vi "Drive Station HUD.vi"() -> ()   [LabVIEW 2018]
uses:
  <vilib>/vision/NI_Vision_Development_Module.lvlib
panel:
  out "Final Image":T1(plugin-control)
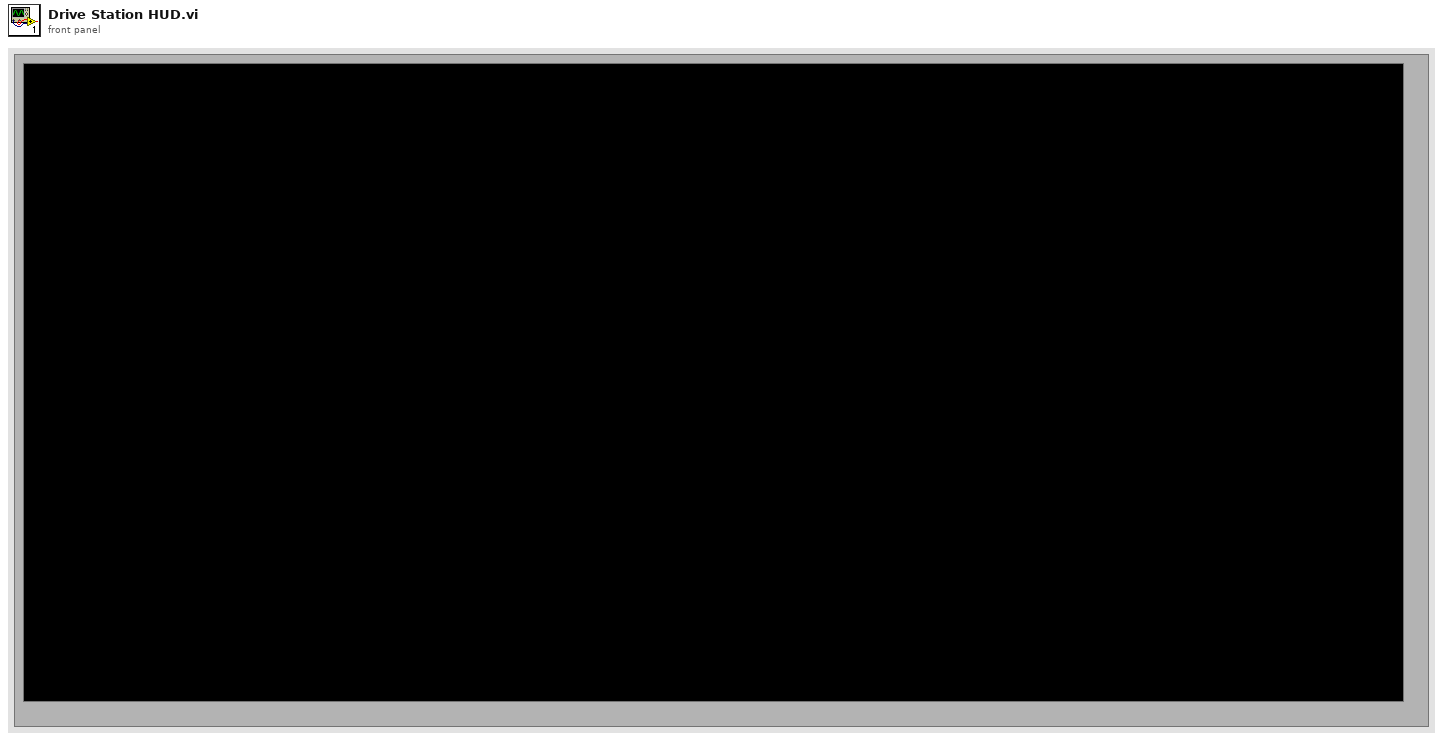
[diagram p1: front panel]
types:
  T1 = typedef "IMAQ Image.ctl" = refnum<image>
  T2 = typedef "Image Type" = u32
  T3 = typedef "LVAllMonitorsDisplayTypeDef.ctl" = cluster{"Bounds":cluster{"Left":i16, "Top":i16, "Right":i16, "Bottom":i16}, "Depth":i16}[]
  T4 = cluster{"Left":i16, "Top":i16, "Right":i16, "Bottom":i16}
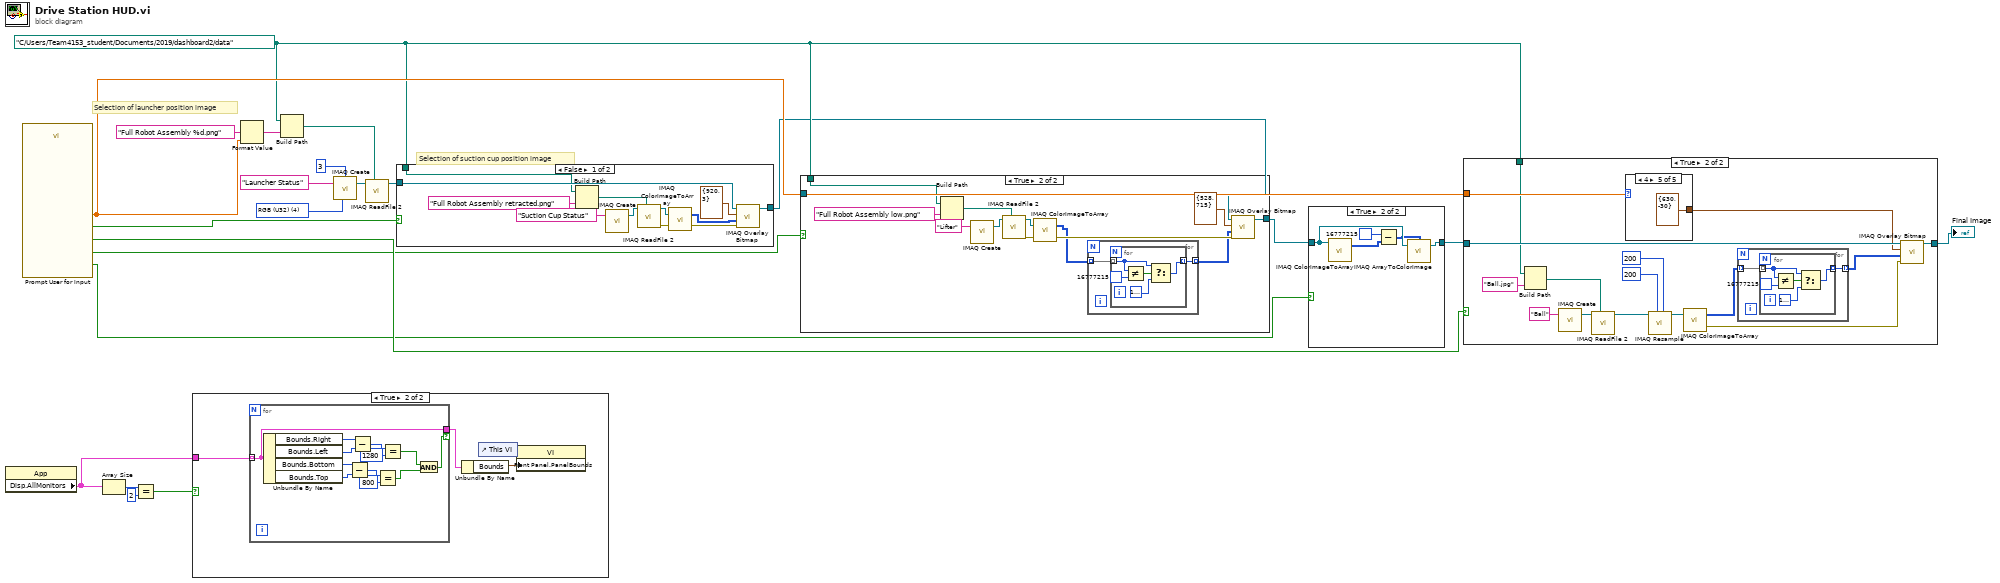
[diagram p0: block diagram]
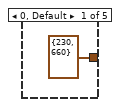
[diagram p6: hidden frame]
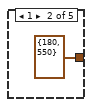
[diagram p7: hidden frame]
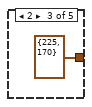
[diagram p8: hidden frame]
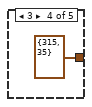
[diagram p9: hidden frame]
diagram:
  w11 = path "C:/Users/Team4153_student/Documents/2019/dashboard2/data"
  w21 = T2 4 items=["Grayscale (U8)", "Grayscale (I16)", "Grayscale (SGL)", "Complex (CSG)", "RGB (U32)", "HSL (U32)", "RGB (U64)", "Grayscale (U16)"] ("Image Type")
  # "Selection of suction cup position image"
  # "Selection of launcher position image"
  n1 = property class="App"() -> ("Disp.AllMonitors"=w1:T3)  [unwired: 2 in, 2 out]
  n2 = call "Prompt User for Input"() -> ("Invert Colors"=w8:bool, "Lifter extended"=w10:bool, "Ball Obtained"=w16:bool, "Suction Cup extended"=w18:bool, "Position of Launcher:"=w14:dbl)  [unwired: 13 in, 2 out]
  n3 = Array Size(array=w1) -> (size(s)=w4:i32)
  n4 = Equal?(x=w4, y=2) -> (x = y?=w2:bool)
  n5 = case shown="True" w2 {
    tunnel: w1 -> [_ w26]
    frame False {
    }
    frame True {
      n6 = for {
        tunnel: w26 -> [w28] mode=indexing
        tunnel: [w28] -> w24 if=w27
        n7 = Unbundle By Name(w28) -> ("Bounds.Right"=w38:i16, "Bounds.Left"=w37:i16, "Bounds.Bottom"=w36:i16, "Bounds.Top"=w35:i16)
        n8 = Subtract(x=w36, y=w35) -> (x-y=w34:i16)
        n9 = Subtract(x=w38, y=w37) -> (x-y=w31:i16)
        n10 = Equal?(x=w34, y=i16 800) -> (x = y?=w29:bool)
        n11 = Equal?(x=w31, y=i16 1280) -> (x = y?=w30:bool)
        n12 = And(x=w30, y=w29) -> (x .and. y?=w27:bool)
      }
      n13 = Unbundle By Name(w24) -> ("Bounds"=w23:T4)
      n14 = control-ref of="This VI"() -> (w25:refnum<vi>)
      n15 = property class="VI"(reference=w25, "Front Panel.PanelBounds"=w23) -> ()  [unwired: 1 in, 2 out]
    }
  }
  n16 = Format Value(format string="Full Robot Assembly %d.png", value (0)=w14) -> (output string=w13:string)  [unwired: 1 in]
  n17 = Build Path(base path=w11, name or relative path=w13) -> (appended path=w12:path)
  n18 = call "IMAQ Create"("Border Size"=3, "Image Name"="Launcher Status", "Image Type"=w21) -> ("New Image"=w20:T1)  [unwired: 2 in, 1 out]
  n19 = call "IMAQ ReadFile 2"("File Path"=w12, "Image"=w20) -> ("Image Out"=w17:T1)  [unwired: 5 in, 4 out]
  n20 = case shown="False" w18 {
    tunnel: w17 -> [w45 w51]
    tunnel: [w48 w51] -> w7
    tunnel: w11 -> [w40 _]
    frame False {
      n21 = Build Path(base path=w40, name or relative path="Full Robot Assembly retracted.png") -> (appended path=w41:path)
      n22 = call "IMAQ Create"("Image Name"="Suction Cup Status") -> ("New Image"=w50:T1)  [unwired: 4 in, 1 out]
      n23 = call "IMAQ ReadFile 2"("File Path"=w41, "Image"=w50) -> ("error out"=w46:errorcluster, "Image Out"=w47:T1)  [unwired: 5 in, 3 out]
      n24 = call "IMAQ ColorImageToArray"("Image"=w47, "error in (no error)"=w46) -> ("Image Pixels (U32)"=w43:u32[][], "error out"=w44:errorcluster)  [unwired: 2 in, 1 out]
      n25 = call "IMAQ Overlay Bitmap"("error in (no error)"=w44, "Bitmap"=w43, "Top Left Point"=cluster{"X":i32, "Y":i32} {"X"=920, "Y"=3}, "Image"=w45) -> ("Image Out"=w48:T1)  [unwired: 6 in, 1 out]
    }
    frame True {
    }
  }
  n26 = case shown="True" w10 {
    tunnel: w7 -> [w52 w60]
    tunnel: [w52 w63] -> w9
    tunnel: w11 -> [_ w57]
    frame False {
    }
    frame True {
      n27 = Build Path(base path=w57, name or relative path="Full Robot Assembly low.png") -> (appended path=w58:path)
      n28 = call "IMAQ Create"("Image Name"="Lifter") -> ("New Image"=w65:T1)  [unwired: 4 in, 1 out]
      n29 = call "IMAQ ReadFile 2"("File Path"=w58, "Image"=w65) -> ("error out"=w61:errorcluster, "Image Out"=w62:T1)  [unwired: 5 in, 3 out]
      n30 = call "IMAQ ColorImageToArray"("Image"=w62, "error in (no error)"=w61) -> ("Image Pixels (U32)"=w54:u32[][], "error out"=w59:errorcluster)  [unwired: 2 in, 1 out]
      n31 = for {
        tunnel: w54 -> [w67] mode=indexing
        tunnel: [w66] -> w53 mode=indexing
        n32 = for {
          tunnel: w67 -> [w70] mode=indexing
          tunnel: [w69] -> w66 mode=indexing
          n33 = Not Equal?(x=w70, y=u32 16777215) -> (x != y?=w71:bool)
          n34 = Select(t=w70, s=w71, f=u32 16777216) -> (s? t:f=w69:u32)
        }
      }
      n35 = call "IMAQ Overlay Bitmap"("error in (no error)"=w59, "Bitmap"=w53, "Top Left Point"=cluster{"X":i32, "Y":i32} {"X"=528, "Y"=715}, "Image"=w60) -> ("Image Out"=w63:T1)  [unwired: 6 in, 1 out]
    }
  }
  n36 = case shown="True" w8 {
    tunnel: [w73 w77] -> w6
    tunnel: w9 -> [w73 w76]
    frame False {
    }
    frame True {
      n37 = call "IMAQ ColorImageToArray"("Image"=w76) -> ("Image Pixels (U32)"=w78:u32[][])  [unwired: 3 in, 2 out]
      n38 = Subtract(x=u32 16777215, y=w78) -> (x-y=w75:u32[][])
      n39 = call "IMAQ ArrayToColorImage"("Image Pixels (U32)"=w75, "Image"=w76) -> ("Image Out"=w77:T1)  [unwired: 3 in, 1 out]
    }
  }
  n40 = case shown="True" w16 {
    tunnel: w6 -> [w79 w95]
    tunnel: [w79 w91] -> w5
    tunnel: w14 -> [_ w90]
    tunnel: w11 -> [_ w80]
    frame False {
    }
    frame True {
      n41 = Build Path(base path=w80, name or relative path="Ball.jpg") -> (appended path=w81:path)
      n42 = call "IMAQ Create"("Image Name"="Ball") -> ("New Image"=w93:T1)  [unwired: 4 in, 1 out]
      n43 = call "IMAQ ReadFile 2"("File Path"=w81, "Image"=w93) -> ("Image Out"=w88:T1)  [unwired: 5 in, 4 out]
      n44 = case shown="4" w90 {
        tunnel: [cluster{"X":i32, "Y":i32} {"X"=230, "Y"=660} ("Top Left Point") cluster{"X":i32, "Y":i32} {"X"=180, "Y"=550} ("Top Left Point") cluster{"X":i32, "Y":i32} {"X"=225, "Y"=170} ("Top Left Point") cluster{"X":i32, "Y":i32} {"X"=315, "Y"=35} ("Top Left Point") cluster{"X":i32, "Y":i32} {"X"=630, "Y"=-30} ("Top Left Point")] -> w89
        frame 0, Default {
        }
        frame 1 {
        }
        frame 2 {
        }
        frame 3 {
        }
        frame 4 {
        }
      }
      n45 = call "IMAQ Resample"("X Resolution"=200, "Y Resolution"=200 ("X Resolution"), "Image Src"=w88) -> ("Image Dst Out"=w87:T1)  [unwired: 7 in, 1 out]
      n46 = call "IMAQ ColorImageToArray"("Image"=w87) -> ("Image Pixels (U32)"=w84:u32[][], "error out"=w92:errorcluster)  [unwired: 3 in, 1 out]
      n47 = for {
        tunnel: w84 -> [w97] mode=indexing
        tunnel: [w96] -> w83 mode=indexing
        n48 = for {
          tunnel: w97 -> [w100] mode=indexing
          tunnel: [w99] -> w96 mode=indexing
          n49 = Not Equal?(x=w100, y=u32 16777215) -> (x != y?=w101:bool)
          n50 = Select(t=w100, s=w101, f=u32 16777216) -> (s? t:f=w99:u32)
        }
      }
      n51 = call "IMAQ Overlay Bitmap"("error in (no error)"=w92, "Bitmap"=w83, "Top Left Point"=w89, "Image"=w95) -> ("Image Out"=w91:T1)  [unwired: 6 in, 1 out]
    }
  }
  "Final Image" <- w5
